vi "Create.vi"(8 "error in (no error)":errorcluster, 11 "I64 array in":i64[](array[numeric])) -> (0 "error out":errorcluster, 3 "Int64Array out":refnum<class "Int64Array.lvclass">)   [LabVIEW 2012, in "MDSplus.lvlib" / "Int64Array.lvclass"]
uses:
  <vilib>/MDSplus/Classes/Data_Class/Array_Class/Int64Array_Class/Int64Array.lvclass
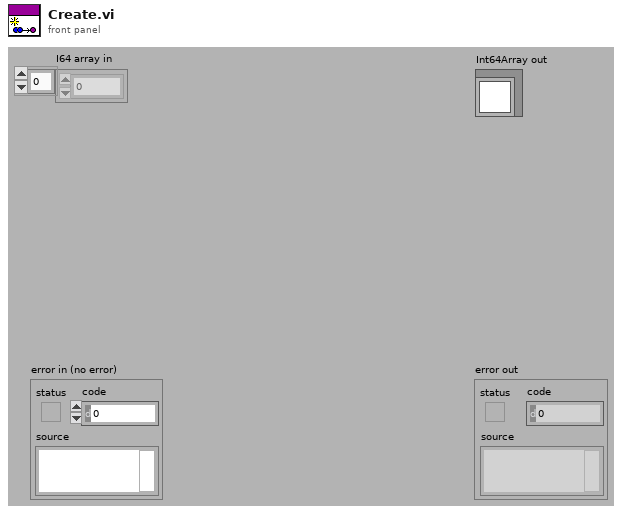
[diagram p1: front panel]
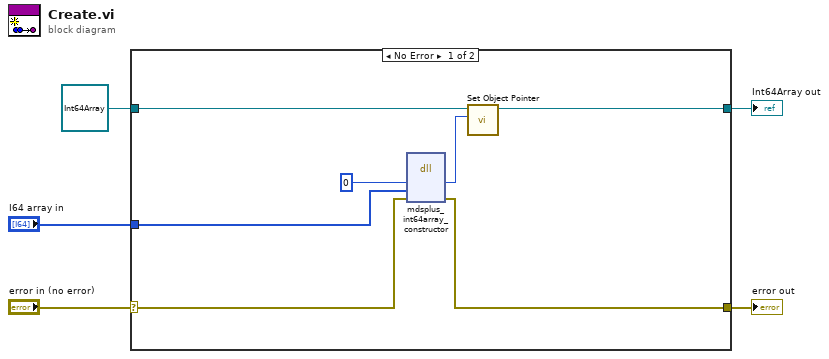
[diagram p0: block diagram]
diagram:
  n1 = case shown="No Error" "error in (no error)" {
    selector: "error in (no error)" -> [w10 w14]
    tunnel: [w6 w14] -> w4
    tunnel: [w8 w13] -> w2
    tunnel: refnum<class "Int64Array.lvclass"> refnum ("Float32 in") -> [w9 w13]
    tunnel: "I64 array in" -> [w7 _]
    frame No Error {
      n2 = dll-call lib="MDSobjectsLVShr" fn="mdsplus_int64array_constructor"("lvInt64ArrayPtrOut"=i64 0 ("lvTreePtr"), "lvLngArrHdlIn"=w7, "error"=w10) -> ("lvInt64ArrayPtrOut"=w11:i64, "error"=w6:errorcluster)  [unwired: 5 in, 2 out]
      n3 = call-dynamic "Set Object Pointer.vi"("Object Pointer"=w11, "Data in"=w9) -> ("Data out"=w8:refnum<class "Int64Array.lvclass">)  [unwired: 9 in]
    }
    frame Error {
    }
  }
  "error out" <- w4
  "Int64Array out" <- w2
